vi "getControlData_distEst.vi"(11 "system matricec path":path=path "C:/Users/arnold/Documents/MATLAB/AFM_MPC/data/MPCControls01.csv") -> (0 "MPC matrices":dbl[][](array[numeric]), 1 "AllMatrix":dbl[](array[numeric]), 2 "QP_params":T2={"maxIter"=0, "nuN"=24, "Ns_mpc"=0, "-beta"=-0.9987945556640625, "beta+1"=1.9987945556640625}, 3 "ControlParams":T3={"umax"=3.0, "NS"=0, "ref_f_VEC"=[0.0, 0.0], "du_max"=0.0}, 4 "ControlMatrices":T1)   [LabVIEW 2017]
doc: "Reads the MPC controller data from a csv file. The format is specified as:\n\n[Ns, ref_f_x, ref_f_y, Nux, Nuy, umax, ]\nbeta, du_max, maxIter, Nmpc, Ns_mpc] \n[AllMatrix(:)' ]"
uses:
  fpga_VIs/fixed-point/typeDefs/FXPControlParams_distEst.ctl
  fpga_VIs/fixed-point/single-axis/fxp_mpc/fgm_pipiline/quadProgParams_pipe.ctl
  controls/ObserverMatrices.ctl
  <vilib>/Utility/file.llb/Read From Spreadsheet File (DBL).vi
panel:
  # "Reads the MPC controller data from a csv file. The format is specified as:\n\n[Ns, ref_f_x, ref_f_y, Nux, Nuy, umax, ]\nbeta, du_max, maxIter, Nmpc, Ns_mpc] \n[AllMatrix(:)'                                              ]"
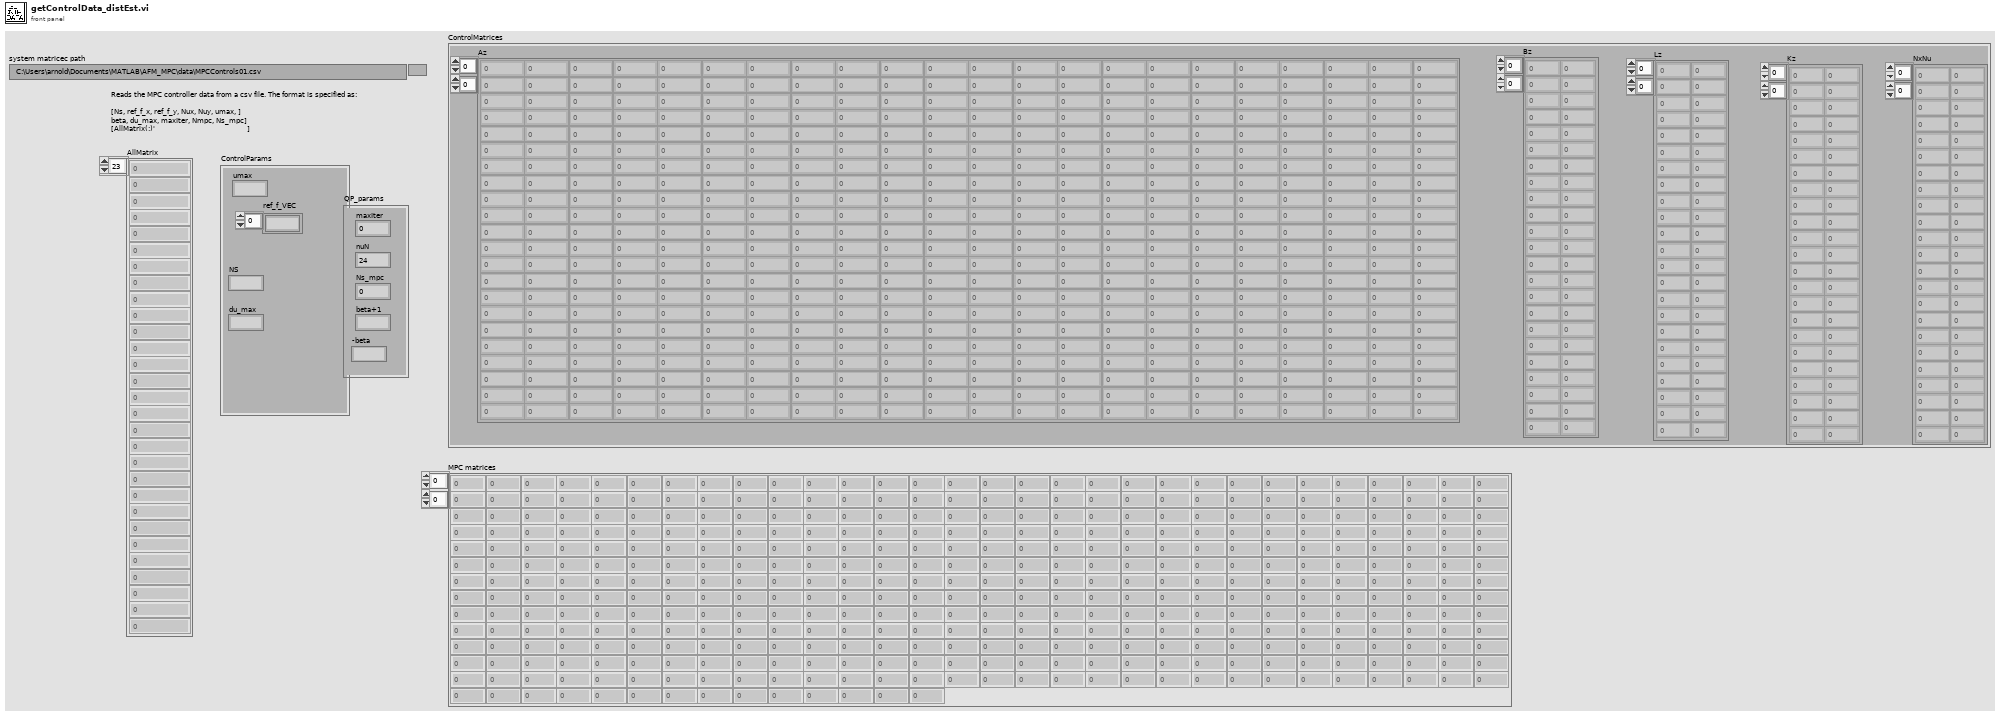
[diagram p1: front panel]
types:
  T1 = typedef "ObserverMatrices.ctl" = cluster{"Az":fxp<+/-,32,4>[][], "Bz":dbl[][], "Lz":dbl[][], "Kz":dbl[][], "NxNu":dbl[][]}
  T2 = typedef "quadProgParams_pipe.ctl" = cluster{"maxIter":u16, "nuN":u16, "Ns_mpc":u16, "-beta":fxp<+/-,18,2>, "beta+1":fxp<+/-,18,2>}
  T3 = typedef "FXPControlParams_distEst.ctl" = cluster{"umax":fxp<+/-,18,5>, "NS":u8, "ref_f_VEC":fxp<+/-,32,5>[], "du_max":fxp<+/-,18,5>}
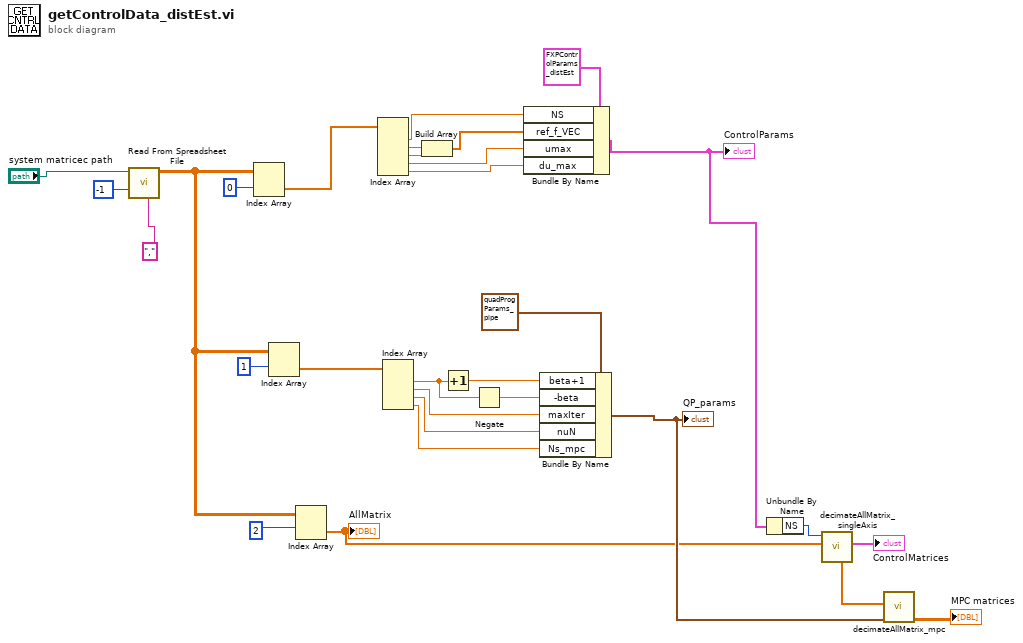
[diagram p0: block diagram]
diagram:
  n1 = call-poly <vilib>:"Read From Spreadsheet File.vi"("delimiter (\\t)"=",", "number of rows (all:-1)"=-1, "file path (dialog if empty)"="system matricec path") -> ("all rows"=w19:dbl[][])  [unwired: 4 in, 4 out]
  n2 = Index Array(array=w19, index (row)=0 ("dimension size")) -> (element=w21:dbl[])  [unwired: 1 in]
  n3 = Index Array(array=w19, index (row)=1 ("dimension size")) -> (element=w27:dbl[])  [unwired: 1 in]
  n4 = Index Array(array=w19, index (row)=2 ("dimension size")) -> (element=w9:dbl[])  [unwired: 1 in]
  "AllMatrix" <- w9
  n5 = Index Array(array=w21) -> (element #1=w23:dbl, element #2=w26:dbl, element #3=w25:dbl, element #4=w5:dbl, element #5=w4:dbl)  [unwired: 5 in]
  n6 = Index Array(array=w27) -> (element #1=w13:dbl, element #2=w3:dbl, element #3=w2:dbl, element #4=w1:dbl)  [unwired: 4 in]
  n7 = Build Array(w26, w25) -> (w22:dbl[])
  n8 = Increment(x=w13) -> (x+1=w15:dbl)
  n9 = Negate(x=w13) -> (-x=w14:dbl)
  n10 = Bundle By Name(cluster=T3 {"umax"=3.0, "NS"=0, "ref_f_VEC"=[0.0, 0.0], "du_max"=0.0} ("ControlParams 2"), "NS"=w23, "ref_f_VEC"=w22, "umax"=w5, "du_max"=w4) -> (w11:T3)
  "ControlParams" <- w11
  n11 = Bundle By Name(cluster=T2 {"maxIter"=0, "nuN"=24, "Ns_mpc"=0, "-beta"=-0.9987945556640625, "beta+1"=1.9987945556640625} ("QP_params 2"), "beta+1"=w15, "-beta"=w14, "maxIter"=w3, "nuN"=w2, "Ns_mpc"=w1) -> (w12:T2)
  "QP_params" <- w12
  n12 = Unbundle By Name(w11) -> ("NS"=w7:u8)
  n13 = call "decimateAllMatrix_singleAxis.vi"("AllMatrix"=w9, "NS"=w7) -> ("ControlMatrices"=→"ControlMatrices":T1, "remaining_array"=w6:dbl[])  [unwired: 8 in]
  n14 = call "decimateAllMatrix_mpc.vi"("QP_params"=w12, "AllMatrix (remainder)"=w6) -> ("MPC matrices"=→"MPC matrices":dbl[][])  [unwired: 9 in]
